vi "ExSubSetCamInSpeFileHeader.vi"(3 "error in (no error)":errorcluster, 4 "Camera Handle":u32, 5 "File Handle":u32) -> (0 "error out":errorcluster, 1 "Camera Handle":u32, 2 "File Handle":u32)   [LabVIEW 2010]
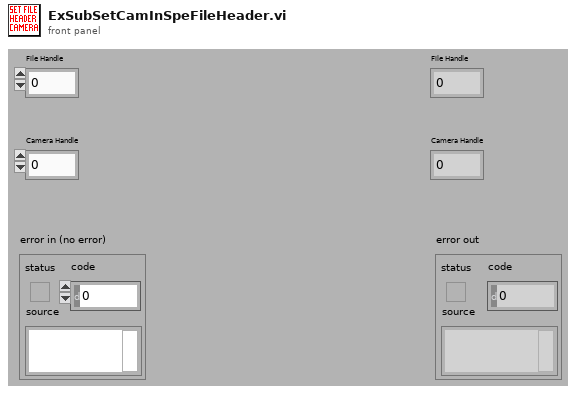
[diagram p1: front panel]
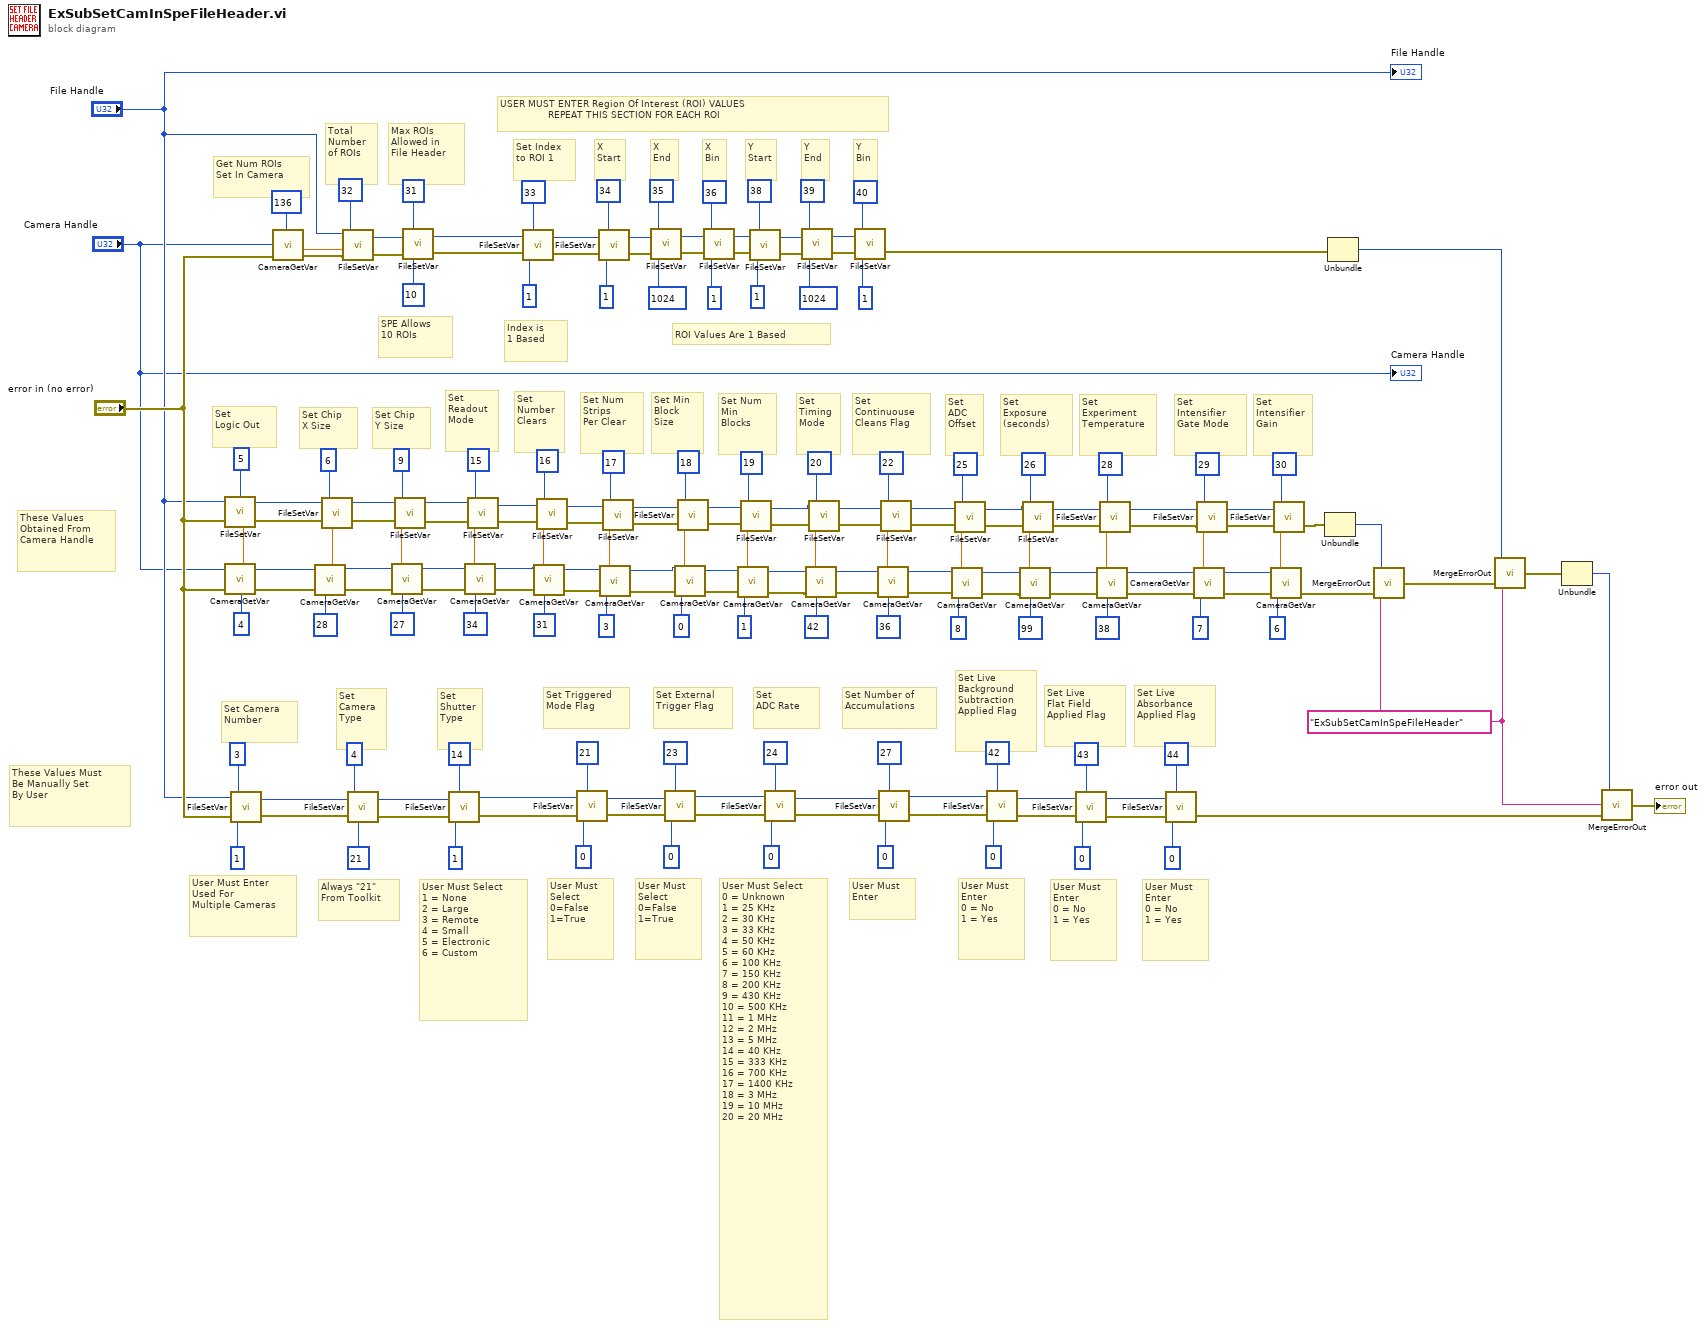
[diagram p0: block diagram]
diagram:
  w1 = "ExSubSetCamInSpeFileHeader"
  # "User Must\nEnter\n0 = No\n1 = Yes"
  # "Set Live\nAbsorbance\nApplied Flag"
  # "User Must\nEnter\n0 = No\n1 = Yes"
  # "Set Live\nFlat Field\nApplied Flag"
  # "User Must\nEnter\n0 = No\n1 = Yes"
  # "Set Live\nBackground\nSubtraction\nApplied Flag"
  # "Set \nIntensifier\nGain"
  # "Set \nIntensifier\nGate Mode"
  # "User Must\nEnter"
  # "Set Number of\nAccumulations"
  # "Set \nExperiment\nTemperature"
  # "Set \nExposure\n(seconds)"
  # "Set\nADC\nOffset"
  # "These Values Must\nBe Manually Set\nBy User"
  # "These Values\nObtained From\nCamera Handle"
  # "User Must Enter\nUsed For\nMultiple Cameras"
  # "Set Camera\nNumber"
  # "User Must Select\n0 = Unknown\n1 = 25 KHz\n2 = 30 KHz\n3 = 33 KHz\n4 = 50 KHz\n5 = 60 KHz\n6 = 100 KHz\n7 = 150 KHz\n8 = 200 KHz\n9 = 430 KHz\n10 = 500 KHz\n11 = 1 MHz\n12 = 2 MHz\n13 = 5 MHz\n14 = 40 KHz\n15 = 333 KHz\n16 = 700 KHz\n17 = 1400 KHz\n18 = 3 MHz\n19 = 10 MHz\n20 = 20 MHz"
  # "Set\nADC Rate"
  # "Set \nContinuouse\nCleans Flag"
  # "Set \nTiming\nMode"
  # "User Must\nSelect\n0=False\n1=True"
  # "Set External\nTrigger Flag"
  # "Set Num\nMin\nBlocks"
  # "Set Min\nBlock\nSize"
  # "Set Num\nStrips\nPer Clear"
  # "Set\nNumber\nClears"
  # "Set\nReadout\nMode"
  # "User Must\nSelect\n0=False\n1=True"
  # "Set Triggered\nMode Flag"
  # "User Must Select\n1 = None\n2 = Large\n3 = Remote\n4 = Small\n5 = Electronic\n6 = Custom"
  # "Set\nShutter\nType"
  # "Always \"21\"\nFrom Toolkit"
  # "Set\nCamera\nType"
  # "Set Chip\nY Size"
  # "Set Chip\nX Size"
  # "Set\nLogic Out"
  # "SPE Allows\n10 ROIs"
  # "Max ROIs\nAllowed in\nFile Header"
  # "Get Num ROIs\nSet In Camera"
  # "USER MUST ENTER Region Of Interest (ROI) VALUES\n                REPEAT THIS SECTION FOR EACH ROI"
  # "Y\nBin"
  # "Y\nEnd"
  # "Y\nStart"
  # "ROI Values Are 1 Based"
  # "X\nBin"
  # "X\nEnd"
  # "X\nStart"
  # "Index is\n1 Based"
  # "Set Index\nto ROI 1"
  # "Total\nNumber\nof ROIs"
  n1 = call <userlib>:"CameraGetVar.vi"("error in"="error in (no error)", "Parameter ID"=4, "Camera Handle"="Camera Handle") -> ("error out"=w141:errorcluster, "Value"=w151:dbl, "Camera Handle"=w143:u32)
  n2 = call <userlib>:"FileSetVar.vi"("error in"="error in (no error)", "Value"=w151, "Parameter ID"=5, "File Handle"="File Handle") -> ("error out"=w139:errorcluster, "File Handle"=w148:u32)
  n3 = call <userlib>:"FileSetVar.vi"("error in"="error in (no error)", "Value"=1, "Parameter ID"=3, "File Handle"="File Handle") -> ("error out"=w68:errorcluster, "File Handle"=w66:u32)
  n4 = call <userlib>:"CameraGetVar.vi"("error in"="error in (no error)", "Parameter ID"=136, "Camera Handle"="Camera Handle") -> ("error out"=w160:errorcluster, "Value"=w161:dbl)  [unwired: 1 out]
  n5 = call <userlib>:"CameraGetVar.vi"("error in"=w141, "Parameter ID"=28, "Camera Handle"=w143) -> ("error out"=w140:errorcluster, "Value"=w138:dbl, "Camera Handle"=w142:u32)
  n6 = call <userlib>:"FileSetVar.vi"("error in"=w139, "Value"=w138, "Parameter ID"=6, "File Handle"=w148) -> ("error out"=w146:errorcluster, "File Handle"=w147:u32)
  n7 = call <userlib>:"FileSetVar.vi"("error in"=w160, "Value"=w161, "Parameter ID"=32, "File Handle"="File Handle") -> ("error out"=w154:errorcluster, "File Handle"=w158:u32)
  n8 = call <userlib>:"FileSetVar.vi"("error in"=w68, "Value"=21, "Parameter ID"=4, "File Handle"=w66) -> ("error out"=w120:errorcluster, "File Handle"=w124:u32)
  n9 = call <userlib>:"CameraGetVar.vi"("error in"=w140, "Parameter ID"=27, "Camera Handle"=w142) -> ("error out"=w125:errorcluster, "Value"=w137:dbl, "Camera Handle"=w126:u32)
  n10 = call <userlib>:"FileSetVar.vi"("error in"=w146, "Value"=w137, "Parameter ID"=9, "File Handle"=w147) -> ("error out"=w127:errorcluster, "File Handle"=w128:u32)
  n11 = call <userlib>:"FileSetVar.vi"("error in"=w154, "Value"=10, "Parameter ID"=31, "File Handle"=w158) -> ("error out"=w156:errorcluster, "File Handle"=w157:u32)
  n12 = call <userlib>:"FileSetVar.vi"("error in"=w120, "Value"=1, "Parameter ID"=14, "File Handle"=w124) -> ("error out"=w122:errorcluster, "File Handle"=w123:u32)
  n13 = call <userlib>:"CameraGetVar.vi"("error in"=w125, "Parameter ID"=34, "Camera Handle"=w126) -> ("error out"=w95:errorcluster, "Value"=w129:dbl, "Camera Handle"=w99:u32)
  n14 = call <userlib>:"FileSetVar.vi"("error in"=w127, "Value"=w129, "Parameter ID"=15, "File Handle"=w128) -> ("error out"=w103:errorcluster, "File Handle"=w107:u32)
  n15 = call <userlib>:"FileSetVar.vi"("error in"=w156, "Value"=1, "Parameter ID"=33, "File Handle"=w157) -> ("error out"=w177:errorcluster, "File Handle"=w180:u32)
  n16 = call <userlib>:"CameraGetVar.vi"("error in"=w95, "Parameter ID"=31, "Camera Handle"=w99) -> ("error out"=w94:errorcluster, "Value"=w117:dbl, "Camera Handle"=w98:u32)
  n17 = call <userlib>:"FileSetVar.vi"("error in"=w103, "Value"=w117, "Parameter ID"=16, "File Handle"=w107) -> ("error out"=w102:errorcluster, "File Handle"=w106:u32)
  n18 = call <userlib>:"FileSetVar.vi"("error in"=w122, "Value"=0, "Parameter ID"=21, "File Handle"=w123) -> ("error out"=w74:errorcluster, "File Handle"=w75:u32)
  n19 = call <userlib>:"FileSetVar.vi"("error in"=w177, "Value"=1, "Parameter ID"=34, "File Handle"=w180) -> ("error out"=w176:errorcluster, "File Handle"=w179:u32)
  n20 = call <userlib>:"CameraGetVar.vi"("error in"=w94, "Parameter ID"=3, "Camera Handle"=w98) -> ("error out"=w93:errorcluster, "Value"=w114:dbl, "Camera Handle"=w97:u32)
  n21 = call <userlib>:"FileSetVar.vi"("error in"=w102, "Value"=w114, "Parameter ID"=17, "File Handle"=w106) -> ("error out"=w101:errorcluster, "File Handle"=w105:u32)
  n22 = call <userlib>:"FileSetVar.vi"("error in"=w176, "Value"=1024, "Parameter ID"=35, "File Handle"=w179) -> ("error out"=w175:errorcluster, "File Handle"=w178:u32)
  n23 = call <userlib>:"FileSetVar.vi"("error in"=w74, "Value"=0, "Parameter ID"=23, "File Handle"=w75) -> ("error out"=w64:errorcluster, "File Handle"=w65:u32)
  n24 = call <userlib>:"CameraGetVar.vi"("error in"=w93, "Parameter ID"=0, "Camera Handle"=w97) -> ("error out"=w92:errorcluster, "Value"=w111:dbl, "Camera Handle"=w96:u32)
  n25 = call <userlib>:"FileSetVar.vi"("error in"=w101, "Value"=w111, "Parameter ID"=18, "File Handle"=w105) -> ("error out"=w100:errorcluster, "File Handle"=w104:u32)
  n26 = call <userlib>:"FileSetVar.vi"("error in"=w175, "Value"=1, "Parameter ID"=36, "File Handle"=w178) -> ("error out"=w163:errorcluster, "File Handle"=w164:u32)
  n27 = call <userlib>:"CameraGetVar.vi"("error in"=w92, "Parameter ID"=1, "Camera Handle"=w96) -> ("error out"=w77:errorcluster, "Value"=w108:dbl, "Camera Handle"=w79:u32)
  n28 = call <userlib>:"FileSetVar.vi"("error in"=w100, "Value"=w108, "Parameter ID"=19, "File Handle"=w104) -> ("error out"=w81:errorcluster, "File Handle"=w83:u32)
  n29 = call <userlib>:"FileSetVar.vi"("error in"=w163, "Value"=1, "Parameter ID"=38, "File Handle"=w164) -> ("error out"=w166:errorcluster, "File Handle"=w168:u32)
  n30 = call <userlib>:"FileSetVar.vi"("error in"=w64, "Value"=0, "Parameter ID"=24, "File Handle"=w65) -> ("error out"=w39:errorcluster, "File Handle"=w40:u32)
  n31 = call <userlib>:"FileSetVar.vi"("error in"=w166, "Value"=1024, "Parameter ID"=39, "File Handle"=w168) -> ("error out"=w165:errorcluster, "File Handle"=w167:u32)
  n32 = call <userlib>:"CameraGetVar.vi"("error in"=w77, "Parameter ID"=42, "Camera Handle"=w79) -> ("error out"=w76:errorcluster, "Value"=w87:dbl, "Camera Handle"=w78:u32)
  n33 = call <userlib>:"FileSetVar.vi"("error in"=w81, "Value"=w87, "Parameter ID"=20, "File Handle"=w83) -> ("error out"=w80:errorcluster, "File Handle"=w82:u32)
  n34 = call <userlib>:"FileSetVar.vi"("error in"=w165, "Value"=1, "Parameter ID"=40, "File Handle"=w167) -> ("error out"=w6:errorcluster)  [unwired: 1 out]
  n35 = call <userlib>:"CameraGetVar.vi"("error in"=w76, "Parameter ID"=36, "Camera Handle"=w78) -> ("error out"=w43:errorcluster, "Value"=w84:dbl, "Camera Handle"=w44:u32)
  n36 = call <userlib>:"FileSetVar.vi"("error in"=w39, "Value"=0, "Parameter ID"=27, "File Handle"=w40) -> ("error out"=w15:errorcluster, "File Handle"=w18:u32)
  n37 = call <userlib>:"FileSetVar.vi"("error in"=w80, "Value"=w84, "Parameter ID"=22, "File Handle"=w82) -> ("error out"=w45:errorcluster, "File Handle"=w46:u32)
  n38 = call <userlib>:"CameraGetVar.vi"("error in"=w43, "Parameter ID"=8, "Camera Handle"=w44) -> ("error out"=w48:errorcluster, "Value"=w61:dbl, "Camera Handle"=w50:u32)
  n39 = call <userlib>:"FileSetVar.vi"("error in"=w45, "Value"=w61, "Parameter ID"=25, "File Handle"=w46) -> ("error out"=w52:errorcluster, "File Handle"=w54:u32)
  n40 = call <userlib>:"FileSetVar.vi"("error in"=w15, "Value"=0, "Parameter ID"=42, "File Handle"=w18) -> ("error out"=w14:errorcluster, "File Handle"=w17:u32)
  n41 = call <userlib>:"CameraGetVar.vi"("error in"=w48, "Parameter ID"=99, "Camera Handle"=w50) -> ("error out"=w47:errorcluster, "Value"=w58:dbl, "Camera Handle"=w49:u32)
  n42 = call <userlib>:"FileSetVar.vi"("error in"=w52, "Value"=w58, "Parameter ID"=26, "File Handle"=w54) -> ("error out"=w51:errorcluster, "File Handle"=w53:u32)
  n43 = call <userlib>:"FileSetVar.vi"("error in"=w14, "Value"=0, "Parameter ID"=43, "File Handle"=w17) -> ("error out"=w13:errorcluster, "File Handle"=w16:u32)
  n44 = call <userlib>:"CameraGetVar.vi"("error in"=w47, "Parameter ID"=38, "Camera Handle"=w49) -> ("error out"=w25:errorcluster, "Value"=w55:dbl, "Camera Handle"=w26:u32)
  n45 = call <userlib>:"FileSetVar.vi"("error in"=w51, "Value"=w55, "Parameter ID"=28, "File Handle"=w53) -> ("error out"=w27:errorcluster, "File Handle"=w28:u32)
  n46 = call <userlib>:"FileSetVar.vi"("error in"=w13, "Value"=0, "Parameter ID"=44, "File Handle"=w16) -> ("error out"=w8:errorcluster)  [unwired: 1 out]
  n47 = call <userlib>:"CameraGetVar.vi"("error in"=w25, "Parameter ID"=7, "Camera Handle"=w26) -> ("error out"=w29:errorcluster, "Value"=w36:dbl, "Camera Handle"=w30:u32)
  n48 = call <userlib>:"FileSetVar.vi"("error in"=w27, "Value"=w36, "Parameter ID"=29, "File Handle"=w28) -> ("error out"=w31:errorcluster, "File Handle"=w32:u32)
  n49 = call <userlib>:"CameraGetVar.vi"("error in"=w29, "Parameter ID"=6, "Camera Handle"=w30) -> ("error out"=w11:errorcluster, "Value"=w33:dbl)  [unwired: 1 out]
  n50 = call <userlib>:"FileSetVar.vi"("error in"=w31, "Value"=w33, "Parameter ID"=30, "File Handle"=w32) -> ("error out"=w10:errorcluster)  [unwired: 1 out]
  n51 = Unbundle(w10) -> ("code"=w9:i32)  [unwired: 2 out]
  n52 = Unbundle(w6) -> ("code"=w5:i32)  [unwired: 2 out]
  n53 = call <userlib>:"MergeErrorOut.vi"("error in"=w11, "Fucntion Name"=w1, "ErrorCode"=w9) -> ("error out"=w4:errorcluster)
  n54 = call <userlib>:"MergeErrorOut.vi"("error in"=w4, "Fucntion Name"=w1, "ErrorCode"=w5) -> ("error out"=w3:errorcluster)
  n55 = Unbundle(w3) -> ("code"=w2:i32)  [unwired: 2 out]
  n56 = call <userlib>:"MergeErrorOut.vi"("error in"=w8, "Fucntion Name"=w1, "ErrorCode"=w2) -> ("error out"=→"error out":errorcluster)
  "File Handle" <- "File Handle"
  "Camera Handle" <- "Camera Handle"
